vi "vision processing.vi"(0 "Image In":T1, 1 "error in (no error)":errorcluster) -> (2 "error out":errorcluster, 3 "height":dbl, 4 "area":dbl, 5 "x":dbl, 6 "y":dbl, 7 "width":dbl)   [LabVIEW 2011]
uses:
  <vilib>/vision/Image Controls.llb/IMAQ Image.ctl
  fg_typedef.ctl
  <vilib>/vision/NI_Vision_Development_Module.lvlib
panel:
  out "Image Out":T1
  out "error out":errorcluster
  out "Number of Particles Found":i32
  out "Image Out":T1
  out "Number of Hoops Found":i32
  # "0  center of mass x\n1  center of mass y\n2  first pixel x\n3  first pixel y\n4  bounding rect left\n5  bounding rect top\n6  bounding rect right\n7  bounding rect bottom\n8 max feret diameter start x\n9  max feret diameter start y\n10 max feret diameter end x\n11 max feret diameter end y\n12 max horiz segment length left\n13 max horiz segment length right\n14 max horiz segment length row\n15 bounding rect width \n16 bounding rect height\n17 bounding rect diagional\n..\n33 area"
  # "13'3\"\n3'9\""
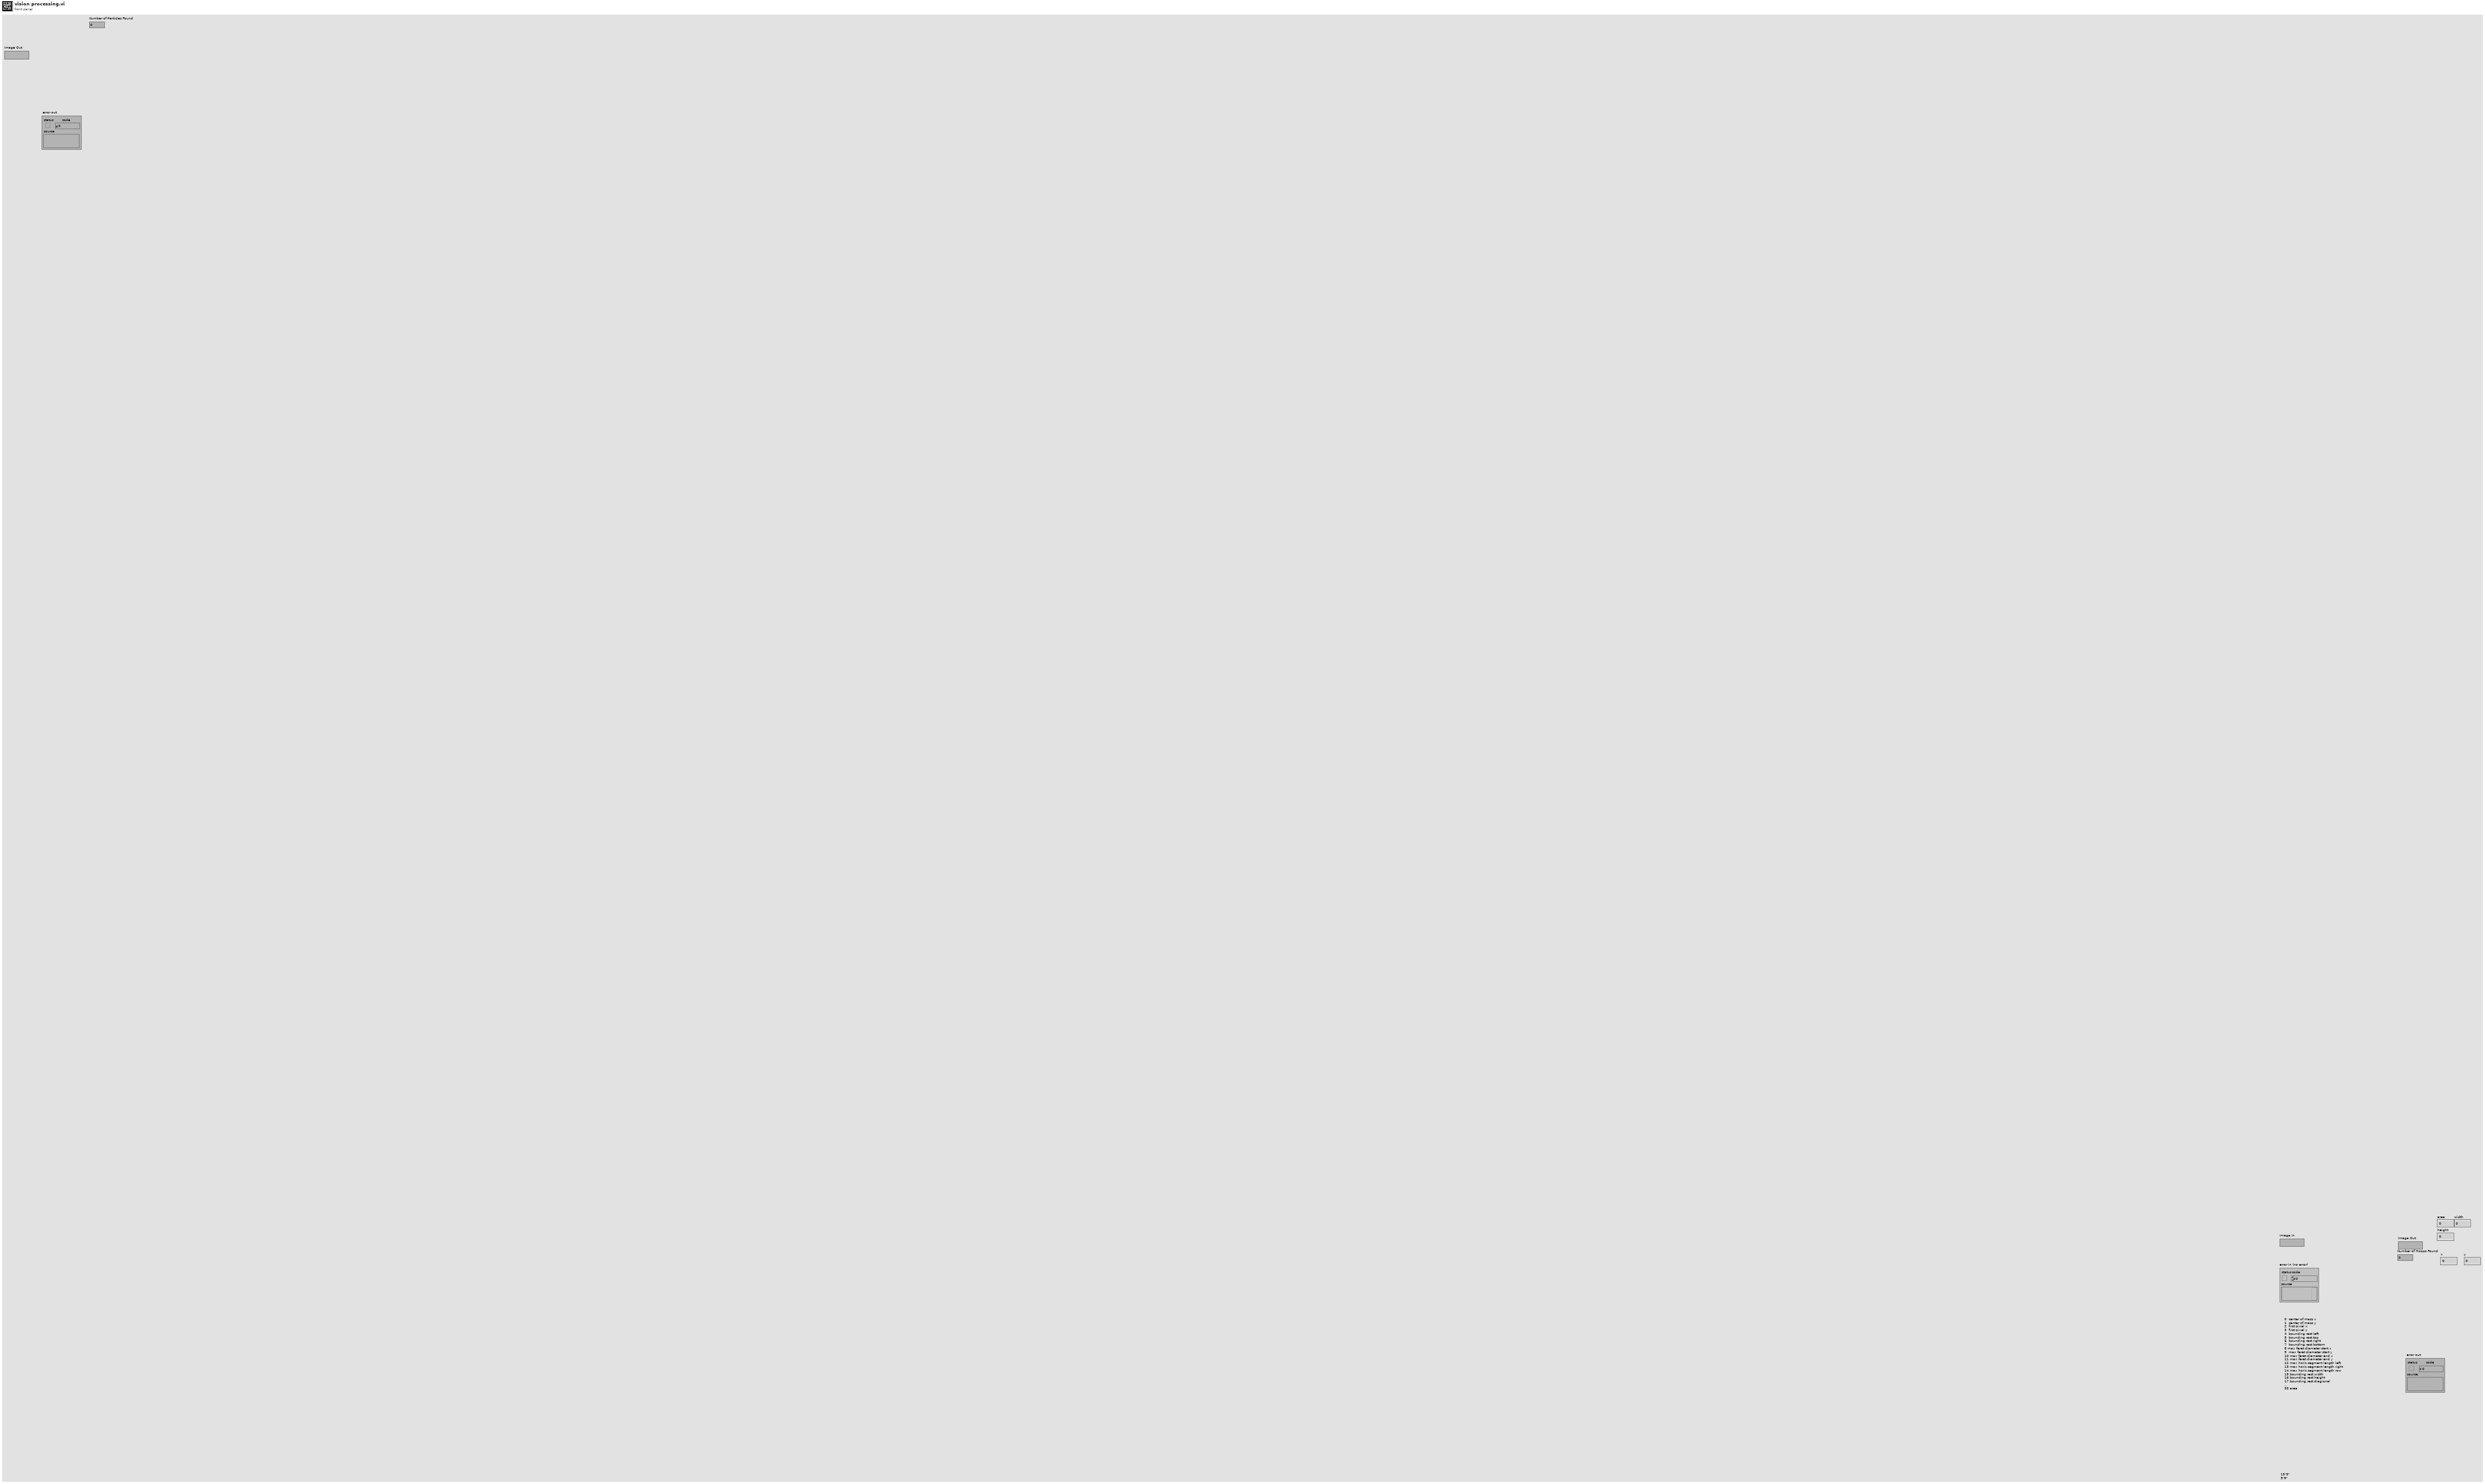
[diagram p1: front panel]
types:
  T1 = typedef "IMAQ Image.ctl" = refnum<image>
  T2 = typedef "Image Type" = u32
  T3 = typedef "fg_typedef.ctl" = enum16{"Get", "Set"}
  T4 = enum32{"AutoM", "Close", "Dilate", "Erode", "Gradient", "Gradient out", "Gradient in", "Hit miss", "Open", "PClose", "POpen", "Thick", "Thin"}
  T5 = cluster{"Brightness":sgl, "Contrast":sgl, "Gamma":sgl}
  T6 = cluster{"Measurement Parameter":i32, "Range Lower Value":dbl, "Range Upper Value":dbl, "Range":bool, "Measurement Type":bool}[]
  T7 = typedef "Particle Parameters" = i32
  T8 = typedef "WPI_DigitalInputDevRef.ctl" = cluster{"DevStatus":errorcluster, "DIO Channel":T9, "Digital Module":T10}
  T9 = typedef "FPGA_DIOChannel.ctl" = enum8{"DIO 1", "DIO 2", "DIO 3", "DIO 4", "DIO 5", "DIO 6", "DIO 7", "DIO 8", "DIO 9", "DIO 10", "DIO 11", "DIO 12", "DIO 13", "DIO 14", "Invalid"}
  T10 = typedef "FPGA_TypedefDigitalModule.ctl" = enum16{"Digital Module 1", "Digital Module 2"}
  T11 = cluster{"Numeric":dbl, "Numeric":dbl, "Numeric":dbl, "Numeric":dbl}
  T12 = cluster{"Numeric":i32, "Numeric":i32, "Numeric":i32, "Numeric":i32}
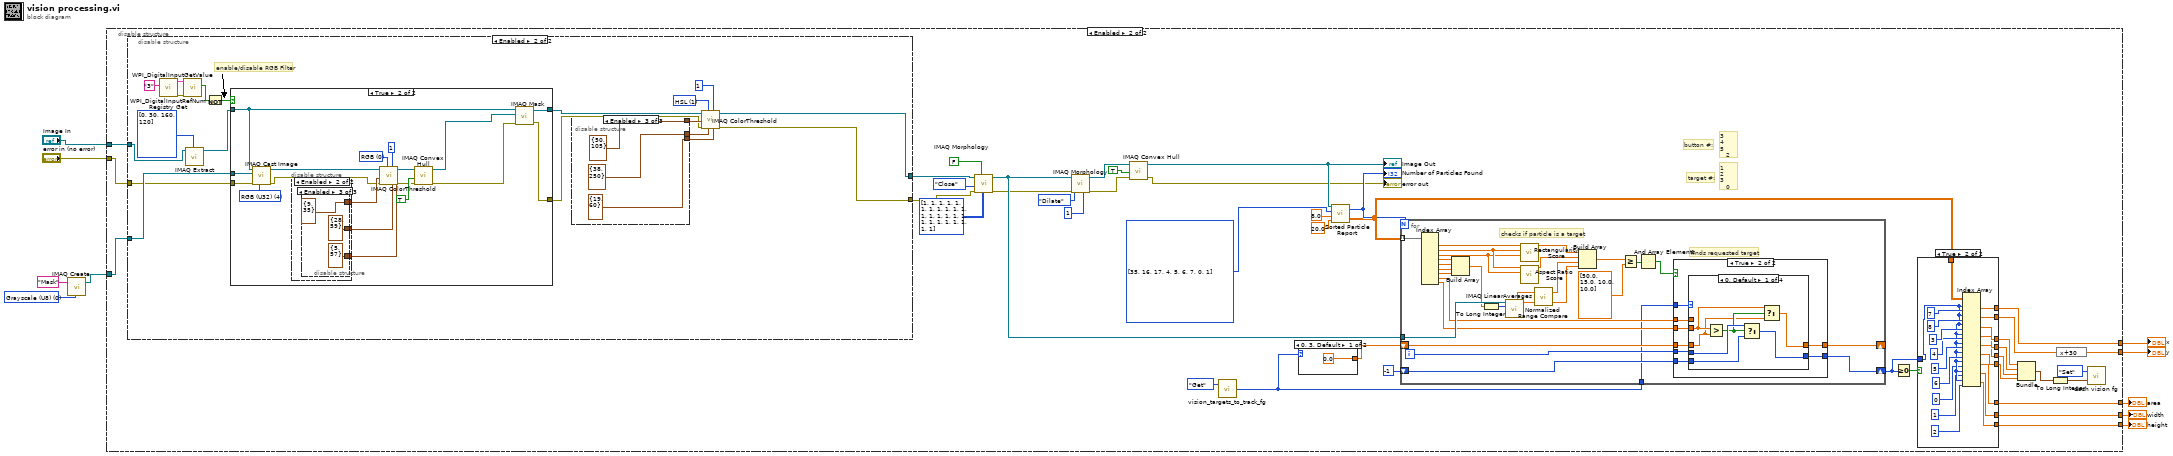
[diagram p0: block diagram]
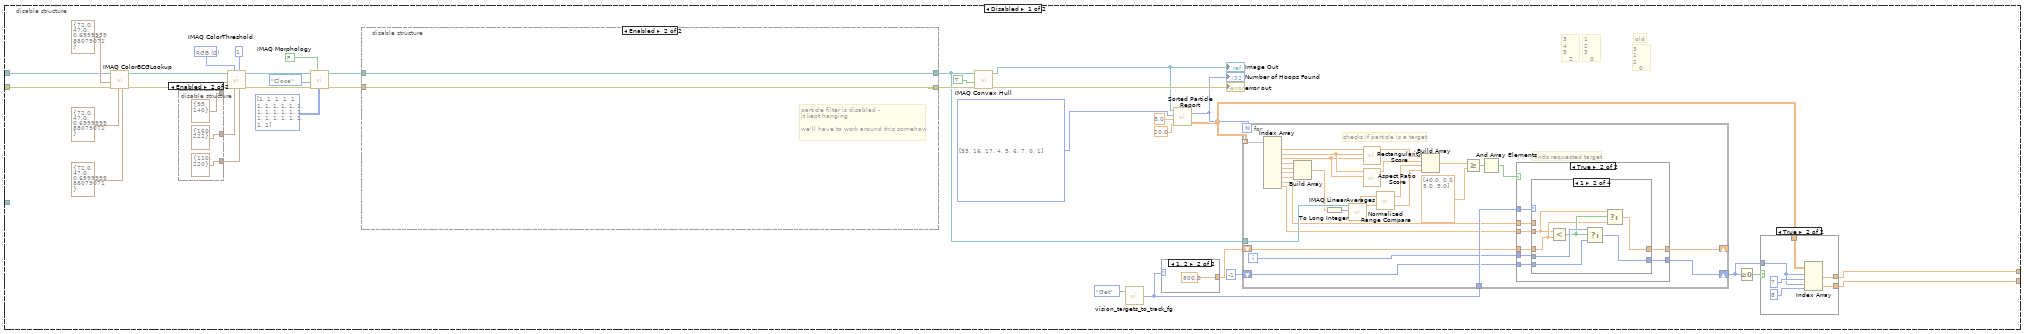
[diagram p2: hidden frame]
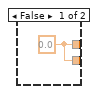
[diagram p3: hidden frame]
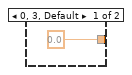
[diagram p4: hidden frame]
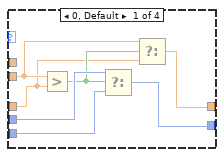
[diagram p6: hidden frame]
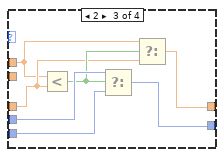
[diagram p7: hidden frame]
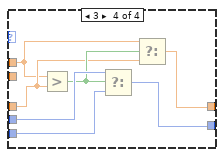
[diagram p8: hidden frame]
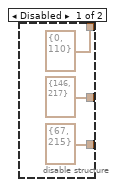
[diagram p9: hidden frame]
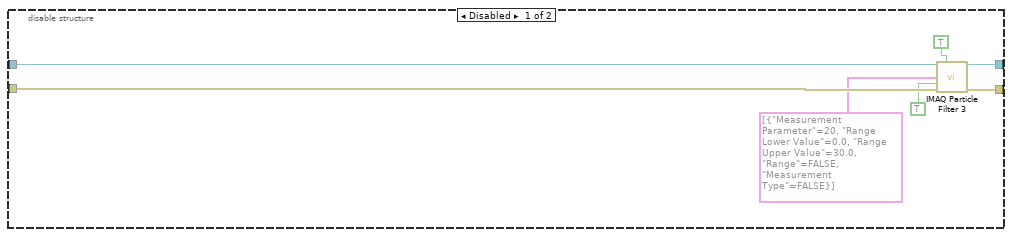
[diagram p10: hidden frame]
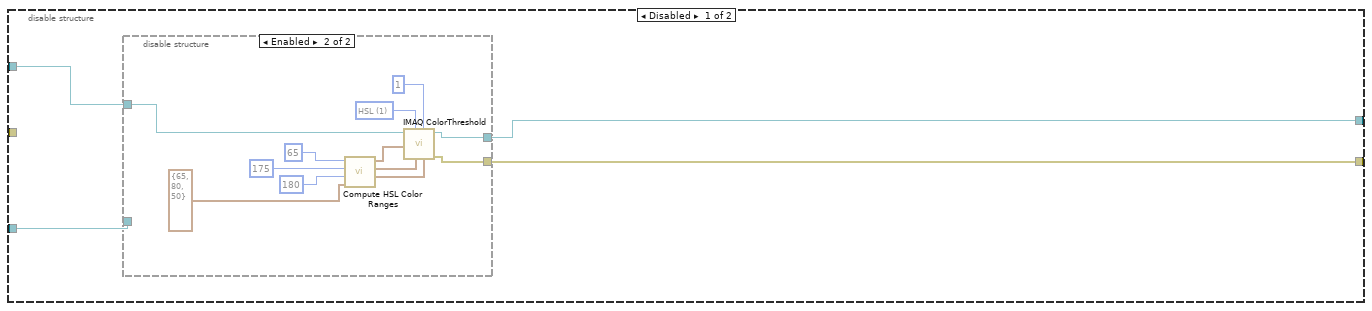
[diagram p11: hidden frame]
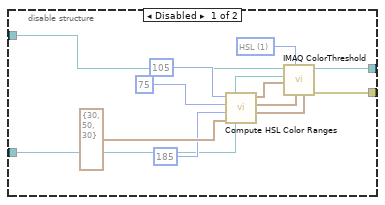
[diagram p12: hidden frame]
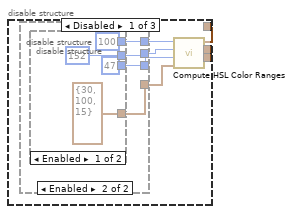
[diagram p13: hidden frame]
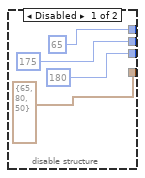
[diagram p14: hidden frame]
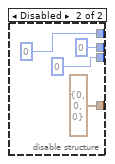
[diagram p15: hidden frame]
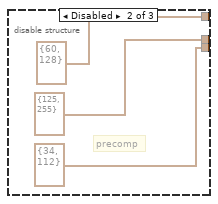
[diagram p16: hidden frame]
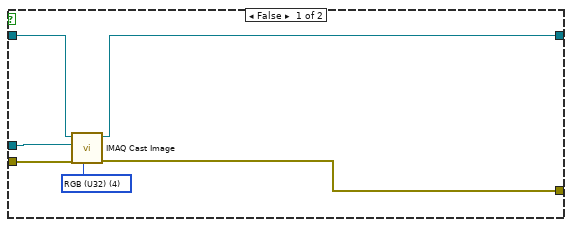
[diagram p17: hidden frame]
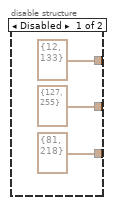
[diagram p18: hidden frame]
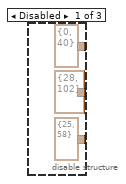
[diagram p19: hidden frame]
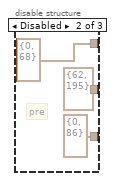
[diagram p20: hidden frame]
diagram:
  w7 = T2 0 items=["Grayscale (U8)", "Grayscale (I16)", "Grayscale (SGL)", "Complex (CSG)", "RGB (U32)", "HSL (U32)", "RGB (U64)", "Grayscale (U16)"] ("Image Type")
  n1 = call "IMAQ Create"("Image Name"="Mask", "Image Type"=w7) -> ("New Image"=w6:T1)  [unwired: 2 in, 2 out]
  n2 = disable-structure shown="Enabled" {
    disable-tunnel: "error in (no error)" -> [w28 w143]
    disable-tunnel: "Image In" -> [w27 w165]
    disable-tunnel: [w13 w162] -> w5
    disable-tunnel: [w12 w139] -> w4
    disable-tunnel: w6 -> [_ w144]
    disable-tunnel: [_ w142] -> w3
    disable-tunnel: [_ w141] -> w2
    disable-tunnel: [_ w140] -> w1
    frame Disabled {
      w20 = T7[] [35, 16, 17, 4, 5, 6, 7, 0, 1] items=["Center of Mass X", "Center of Mass Y", "First Pixel X", "First Pixel Y", "Bounding Rect Left", "Bounding Rect Top", "Bounding Rect Right", "Bounding Rect Bottom", "Max Feret Diameter Start X", "Max Feret Diameter Start Y", "Max Feret Diameter End X", "Max Feret Diameter End Y", "Max Horiz. Segment Length Left", "Max Horiz. Segment Length Right", "Max Horiz. Segment Length Row", "-", "Bounding Rect Width", "Bounding Rect Height", "Bounding Rect Diagonal", "Perimeter", "Convex Hull Perimeter", "Holes' Perimeter", "Max Feret Diameter", "Equivalent Ellipse Major Axis", "Equivalent Ellipse Minor Axis", "Equivalent Ellipse Minor Axis (Feret)", "Equivalent Rect Long Side", "Equivalent Rect Short Side", "Equivalent Rect Diagonal", "Equivalent Rect Short Side (Feret)", "Average Horiz. Segment Length", "Average Vert. Segment Length", "Hydraulic Radius", "Waddel Disk Diameter", "-", "Area", "Holes' Area", "Particle & Holes' Area", "Convex Hull Area", "Image Area", "-", "Number of Holes", "Number of Horiz. Segments", "Number of Vert. Segments", "-", "Orientation", "Max Feret Diameter Orientation", "-", "% Area/Image Area", "% Area/(Particle & Holes' Area)", "Ratio of Equivalent Ellipse Axes", "Ratio of Equivalent Rect Sides", "-", "Elongation Factor", "Compactness Factor", "Heywood Circularity Factor", "Type Factor", "-", "Sum X", "Sum Y", "Sum XX", "Sum XY", "Sum YY", "Sum XXX", "Sum XXY", "Sum XYY", "Sum YYY", "-", "Moment of Inertia XX", "Moment of Inertia XY", "Moment of Inertia YY", "Moment of Inertia XXX", "Moment of Inertia XXY", "Moment of Inertia XYY", "Moment of Inertia YYY", "Norm. Moment of Inertia XX", "Norm. Moment of Inertia XY", "Norm. Moment of Inertia YY", "Norm. Moment of Inertia XXX", "Norm. Moment of Inertia XXY", "Norm. Moment of Inertia XYY", "Norm. Moment of Inertia YYY", "Hu Moment 1", "Hu Moment 2", "Hu Moment 3", "Hu Moment 4", "Hu Moment 5", "Hu Moment 6", "Hu Moment 7"] ("Requested Particle Measurements")
      w42 = u16 0 items=["RGB", "HSL", "HSV", "HSI"] ("Color Mode")
      # "old"
      # "1   \n2     3\n   0"
      # "3   \n1     2\n   0"
      # "3   \n4     5\n   2"
      n3 = call "IMAQ ColorBCGLookup"("Blue BCG Values"=T5 {"Brightness"=72.0, "Contrast"=47.0, "Gamma"=0.7}, "Green BCG Values"=T5 {"Brightness"=72.0, "Contrast"=47.0, "Gamma"=0.7}, "error in (no error)"=w28, "Red BCG Values"=T5 {"Brightness"=72.0, "Contrast"=47.0, "Gamma"=0.7}, "Image Src"=w27) -> ("error out"=w47:errorcluster, "Image Dst Out"=w38:T1)  [unwired: 2 in, 3 out]
      n4 = disable-structure shown="Enabled" {
        disable-tunnel: [cluster{"Lower value":i32, "Upper value":i32} {"Lower value"=0, "Upper value"=110} ("Red or Hue Range") cluster{"Lower value":i32, "Upper value":i32} {"Lower value"=95, "Upper value"=140} ("Red or Hue Range")] -> w41
        disable-tunnel: [cluster{"Lower value":i32, "Upper value":i32} {"Lower value"=146, "Upper value"=217} ("Green or Sat Range") cluster{"Lower value":i32, "Upper value":i32} {"Lower value"=160, "Upper value"=222} ("Green or Sat Range")] -> w40
        disable-tunnel: [cluster{"Lower value":i32, "Upper value":i32} {"Lower value"=67, "Upper value"=215} ("Blue or Luma or Val or Inten Range") cluster{"Lower value":i32, "Upper value":i32} {"Lower value"=110, "Upper value"=220} ("Blue or Luma or Val or Inten Range")] -> w39
        frame Disabled {
        }
        frame Enabled {
        }
      }
      n5 = call "IMAQ ColorThreshold"("Blue or Luma or Val or Inten Range"=w39, "Replace Value"=1, "Green or Sat Range"=w40, "Color Mode"=w42, "error in (no error)"=w47, "Red or Hue Range"=w41, "Image Src"=w38) -> ("error out"=w37:errorcluster, "Image Dst Out"=w33:T1)  [unwired: 1 in, 2 out]
      n6 = call "IMAQ Morphology"("Structuring Element"=i32[][] [[1, 1, 1, 1, 1], [1, 1, 1, 1, 1], [1, 1, 1, 1, 1], [1, 1, 1, 1, 1], [1, 1, 1, 1, 1]], "Square/Hexa (Square)"=FALSE, "error in (no error)"=w37, "Operation"=T4."Close", "Image Src"=w33) -> ("error out"=w32:errorcluster, "Image Dst Out"=w30:T1)  [unwired: 2 in, 3 out]
      n7 = disable-structure shown="Enabled" {
        disable-tunnel: w32 -> [w136 w138]
        disable-tunnel: [w133 w138] -> w31
        disable-tunnel: w30 -> [w132 w137]
        disable-tunnel: [w130 w137] -> w26
        frame Disabled {
          n8 = call "IMAQ Particle Filter 3"("Image Src"=w132, "Connectivity 4/8 (8)"=TRUE, "Selection Values"=T6 [{"Measurement Parameter"=20, "Range Lower Value"=0.0, "Range Upper Value"=30.0, "Range"=FALSE, "Measurement Type"=FALSE}], "Keep/Remove Particles (F)"=TRUE ("Keep/Remove Particles"), "error in (no error)"=w136) -> ("Image Dst Out"=w130:T1, "error out"=w133:errorcluster)  [unwired: 4 in, 5 out]
        }
        frame Enabled {
          # "particle filter is disabled - \nit kept hanging\n\nwe'll have to work around this somehow"
        }
      }
      n9 = call "IMAQ Convex Hull"("error in (no error)"=w31, "Connectivity 4/8 (8)"=TRUE, "Image Src"=w26) -> ("error out"=→"error out":errorcluster, "Image Dst Out"=w11:T1)  [unwired: 1 in, 6 out]
      "Image Out" <- w11
      n10 = call "vision_targets_to_track_fg.vi"("Menu (Get)"=fg_typedef."Get") -> ("Output"=w23:i32)  [unwired: 1 in]
      n11 = case shown="1, 2" w23 {
        tunnel: [0.0 ("element") 800.0 ("element")] -> w24
        frame 0, 3, Default {
        }
        frame 1, 2 {
        }
      }
      n12 = call "Sorted Particle Report.vi"("Area Size Limit"=20.0, "Particle Count Limit"=8.0, "Pixel Measurements"=w20, "Image in"=w11) -> ("Sorted Data"=w16:dbl[][], "Particles"=w17:i32)
      "Number of Hoops Found" <- w17
      n13 = for {
        N: w17 -> [_]
        tunnel: w26 -> [w85]
        tunnel: w16 -> [w84] mode=indexing
        tunnel: w23 -> [w74]
        shift-right: [w66] -> _
        shift-left: w24 -> [w69]
        shift-right: [w67] -> w15
        shift-left: -1 -> [w68]
        i -> [w70]
        # "checks if particle is a target"
        # "finds requested target"
        n14 = Index Array(array=w84) -> (element #1=w65:dbl, element #2=w62:dbl, element #3=w61:dbl, element #4=w80:dbl, element #5=w79:dbl, element #6=w78:dbl, element #7=w77:dbl, element #8=w72:dbl, element #9=w73:dbl)  [unwired: 9 in]
        n15 = Build Array(w80, w79, w78, w77) -> (w76:dbl[])
        n16 = To Long Integer(number=w76) -> (32bit integer=w75:i32[])
        n17 = call "IMAQ LinearAverages"("Optional Rectangle"=w75, "Image Src"=w85) -> ("Y Axis Averages"=w57:sgl[], "X Axis Averages"=w58:sgl[])  [unwired: 2 in, 6 out]
        n18 = call "Rectangularity Score.vi"("Height"=w61, "Width"=w62, "Area"=w65) -> ("Score"=w64:dbl)  [unwired: 8 in]
        n19 = call "Aspect Ratio Score.vi"("Height"=w61, "Width"=w62) -> ("Score"=w63:dbl)  [unwired: 9 in]
        n20 = call "Normalized Range Compare.vi"("Y Averages"=w57, "X Averages"=w58) -> ("Y Score"=w59:dbl, "X Score"=w60:dbl)
        n21 = Build Array(w64, w63, w60, w59) -> (w83:dbl[])
        n22 = Greater Or Equal?(x=w83, y=dbl[] [40.0, 0.0, 5.0, 5.0]) -> (x >= y?=w81:bool[])
        n23 = And Array Elements(Boolean array=w81) -> (logical AND=w71:bool)
        n24 = case shown="True" w71 {
          tunnel: w74 -> [_ w95]
          tunnel: w73 -> [_ w94]
          tunnel: w72 -> [_ w93]
          tunnel: w70 -> [_ w92]
          tunnel: w69 -> [w86 w91]
          tunnel: w68 -> [w87 w90]
          tunnel: [w87 w89] -> w67
          tunnel: [w86 w88] -> w66
          frame False {
          }
          frame True {
            n25 = case shown="1" w95 {
              tunnel: w94 -> [w98 w103 _ _]
              tunnel: w93 -> [_ _ w110 w117]
              tunnel: w92 -> [w102 w109 w116 w123]
              tunnel: w91 -> [w97 w105 w112 w119]
              tunnel: w90 -> [w101 w108 w115 w122]
              tunnel: [w100 w107 w114 w121] -> w89
              tunnel: [w96 w104 w111 w118] -> w88
              frame 0, Default {
                n26 = Greater?(x=w98, y=w97) -> (0:w99:bool)
                n27 = Select(t=w102, s=w99, f=w101) -> (s? t:f=w100:i32)
                n28 = Select(t=w98, s=w99, f=w97) -> (s? t:f=w96:dbl)
              }
              frame 1 {
                n29 = Less?(x=w103, y=w105) -> (x < y?=w106:bool)
                n30 = Select(t=w109, s=w106, f=w108) -> (s? t:f=w107:i32)
                n31 = Select(t=w103, s=w106, f=w105) -> (s? t:f=w104:dbl)
              }
              frame 2 {
                n32 = Less?(x=w110, y=w112) -> (x < y?=w113:bool)
                n33 = Select(t=w116, s=w113, f=w115) -> (s? t:f=w114:i32)
                n34 = Select(t=w110, s=w113, f=w112) -> (s? t:f=w111:dbl)
              }
              frame 3 {
                n35 = Greater?(x=w117, y=w119) -> (0:w120:bool)
                n36 = Select(t=w123, s=w120, f=w122) -> (s? t:f=w121:i32)
                n37 = Select(t=w117, s=w120, f=w119) -> (s? t:f=w118:dbl)
              }
            }
          }
        }
      }
      n38 = Greater Or Equal To 0?(x=w15) -> (x >= 0?=w14:bool)
      n39 = case shown="True" w14 {
        tunnel: [w48 w52] -> w13
        tunnel: [w48 w51] -> w12
        tunnel: w16 -> [_ w50]
        tunnel: w15 -> [_ w49]
        frame False {
          w48 = 0.0 ("Numeric")
        }
        frame True {
          n40 = Index Array(array=w50, index (row) #1=w49, index (col) #1=7, index (row) #2=w49, index (col) #2=8) -> (element #1=w52:dbl, element #2=w51:dbl)
        }
      }
    }
    frame Enabled {
      w164 = T7[] [35, 16, 17, 4, 5, 6, 7, 0, 1] items=["Center of Mass X", "Center of Mass Y", "First Pixel X", "First Pixel Y", "Bounding Rect Left", "Bounding Rect Top", "Bounding Rect Right", "Bounding Rect Bottom", "Max Feret Diameter Start X", "Max Feret Diameter Start Y", "Max Feret Diameter End X", "Max Feret Diameter End Y", "Max Horiz. Segment Length Left", "Max Horiz. Segment Length Right", "Max Horiz. Segment Length Row", "-", "Bounding Rect Width", "Bounding Rect Height", "Bounding Rect Diagonal", "Perimeter", "Convex Hull Perimeter", "Holes' Perimeter", "Max Feret Diameter", "Equivalent Ellipse Major Axis", "Equivalent Ellipse Minor Axis", "Equivalent Ellipse Minor Axis (Feret)", "Equivalent Rect Long Side", "Equivalent Rect Short Side", "Equivalent Rect Diagonal", "Equivalent Rect Short Side (Feret)", "Average Horiz. Segment Length", "Average Vert. Segment Length", "Hydraulic Radius", "Waddel Disk Diameter", "-", "Area", "Holes' Area", "Particle & Holes' Area", "Convex Hull Area", "Image Area", "-", "Number of Holes", "Number of Horiz. Segments", "Number of Vert. Segments", "-", "Orientation", "Max Feret Diameter Orientation", "-", "% Area/Image Area", "% Area/(Particle & Holes' Area)", "Ratio of Equivalent Ellipse Axes", "Ratio of Equivalent Rect Sides", "-", "Elongation Factor", "Compactness Factor", "Heywood Circularity Factor", "Type Factor", "-", "Sum X", "Sum Y", "Sum XX", "Sum XY", "Sum YY", "Sum XXX", "Sum XXY", "Sum XYY", "Sum YYY", "-", "Moment of Inertia XX", "Moment of Inertia XY", "Moment of Inertia YY", "Moment of Inertia XXX", "Moment of Inertia XXY", "Moment of Inertia XYY", "Moment of Inertia YYY", "Norm. Moment of Inertia XX", "Norm. Moment of Inertia XY", "Norm. Moment of Inertia YY", "Norm. Moment of Inertia XXX", "Norm. Moment of Inertia XXY", "Norm. Moment of Inertia XYY", "Norm. Moment of Inertia YYY", "Hu Moment 1", "Hu Moment 2", "Hu Moment 3", "Hu Moment 4", "Hu Moment 5", "Hu Moment 6", "Hu Moment 7"] ("Requested Particle Measurements")
      # "target #:"
      # "button #:"
      # "1   \n2     3\n   0"
      # "3   \n4     5\n   2"
      n41 = disable-structure shown="Enabled" {
        disable-tunnel: [w183 w216] -> w176
        disable-tunnel: [w182 w217] -> w175
        disable-tunnel: w165 -> [w181 w209]
        disable-tunnel: w144 -> [w180 w226]
        disable-tunnel: w143 -> [_ w225]
        frame Disabled {
          n42 = disable-structure shown="Enabled" {
            disable-tunnel: [w195 w198] -> w183
            disable-tunnel: [w194 w199] -> w182
            disable-tunnel: w181 -> [w185 w197]
            disable-tunnel: w180 -> [w184 _]
            frame Disabled {
              w193 = u16 1 items=["RGB", "HSL", "HSV", "HSI"] ("Color Mode")
              n43 = call "Compute HSL Color Ranges.vi"("Margins"=cluster{"Hue":i32, "Sat":i32, "Lum":i32} {"Hue"=30, "Sat"=50, "Lum"=30}, "Luminance"=185, "Saturation"=75, "Hue"=105) -> ("Lum Range"=w190:cluster{i32, i32}, "Sat Range"=w191:cluster{i32, i32}, "Hue Range"=w192:cluster{i32, i32})  [unwired: 5 in]
              n44 = call "IMAQ ColorThreshold"("Blue or Luma or Val or Inten Range"=w190, "Green or Sat Range"=w191, "Color Mode"=w193, "Red or Hue Range"=w192, "Image Dst"=w184, "Image Src"=w185) -> ("error out"=w195:errorcluster, "Image Dst Out"=w194:T1)  [unwired: 4 in]
            }
            frame Enabled {
              w201 = u16 1 items=["RGB", "HSL", "HSV", "HSI"] ("Color Mode")
              n45 = call "Compute HSL Color Ranges.vi"("Margins"=cluster{"Hue":i32, "Sat":i32, "Lum":i32} {"Hue"=65, "Sat"=80, "Lum"=50}, "Luminance"=180, "Saturation"=175, "Hue"=65) -> ("Lum Range"=w204:cluster{i32, i32}, "Sat Range"=w203:cluster{i32, i32}, "Hue Range"=w202:cluster{i32, i32})  [unwired: 5 in]
              n46 = call "IMAQ ColorThreshold"("Blue or Luma or Val or Inten Range"=w204, "Replace Value"=1, "Green or Sat Range"=w203, "Color Mode"=w201, "Red or Hue Range"=w202, "Image Src"=w197) -> ("error out"=w198:errorcluster, "Image Dst Out"=w199:T1)  [unwired: 4 in]
            }
          }
        }
        frame Enabled {
          w221 = u16 1 items=["RGB", "HSL", "HSV", "HSI"] ("Color Mode")
          # "enable/disable RGB Filter"
          n47 = call <vilib>:"WPI_DigitalInputRefNum Registry Get.vi"("refnum name"="3") -> ("error out"=w214:errorcluster, "DigitalInputDevRef"=w215:T8)  [unwired: 9 in]
          n48 = call <vilib>:"WPI_DigitalInputGetValue.vi"("error in (no error)"=w214, "DigitalInputDevRef"=w215) -> ("Value"=w212:bool)  [unwired: 7 in, 2 out]
          n49 = call "IMAQ Extract"("Optional Rectangle"=i32[] [0, 30, 160, 120], "Image Src"=w209) -> ("Image Dst Out"=w208:T1)  [unwired: 8 in, 1 out]
          n50 = Not(x=w212) -> (.not. x?=w211:bool)
          n51 = case shown="True" w211 {
            tunnel: [w258 w279] -> w219
            tunnel: w226 -> [w260 w271]
            tunnel: w208 -> [w259 w270]
            tunnel: [w257 w266] -> w218
            tunnel: w225 -> [w256 w263]
            frame False {
              w261 = T2 4 items=["Grayscale (U8)", "Grayscale (I16)", "Grayscale (SGL)", "Complex (CSG)", "RGB (U32)", "HSL (U32)", "RGB (U64)"] ("Image Type")
              n52 = call "IMAQ Cast Image"("Image Type"=w261, "error in (no error)"=w256, "Image Dst"=w260, "Image Src"=w259) -> ("error out"=w257:errorcluster, "Image Dst Out"=w258:T1)  [unwired: 6 in]
            }
            frame True {
              w276 = u16 0 items=["RGB", "HSL", "HSV", "HSI"] ("Color Mode")
              w278 = T2 4 items=["Grayscale (U8)", "Grayscale (I16)", "Grayscale (SGL)", "Complex (CSG)", "RGB (U32)", "HSL (U32)", "RGB (U64)"] ("Image Type")
              n53 = call "IMAQ Cast Image"("Image Type"=w278, "error in (no error)"=w263, "Image Dst"=w271, "Image Src"=w270) -> ("error out"=w264:errorcluster, "Image Dst Out"=w274:T1)  [unwired: 6 in]
              n54 = disable-structure shown="Enabled" {
                disable-tunnel: [cluster{"Lower value":i32, "Upper value":i32} {"Lower value"=12, "Upper value"=133} ("Red or Hue Range") w285] -> w268
                disable-tunnel: [cluster{"Lower value":i32, "Upper value":i32} {"Lower value"=127, "Upper value"=255} ("Green or Sat Range") w284] -> w267
                disable-tunnel: [cluster{"Lower value":i32, "Upper value":i32} {"Lower value"=81, "Upper value"=218} ("Blue or Luma or Val or Inten Range") w283] -> w262
                frame Disabled {
                }
                frame Enabled {
                  n55 = disable-structure shown="Enabled" {
                    disable-tunnel: [cluster{"Lower value":i32, "Upper value":i32} {"Lower value"=0, "Upper value"=40} ("Red or Hue Range") cluster{"Lower value":i32, "Upper value":i32} {"Lower value"=0, "Upper value"=68} ("Red or Hue Range") cluster{"Lower value":i32, "Upper value":i32} {"Lower value"=9, "Upper value"=35} ("Red or Hue Range")] -> w285
                    disable-tunnel: [cluster{"Lower value":i32, "Upper value":i32} {"Lower value"=28, "Upper value"=102} ("Green or Sat Range") cluster{"Lower value":i32, "Upper value":i32} {"Lower value"=62, "Upper value"=195} ("Green or Sat Range") cluster{"Lower value":i32, "Upper value":i32} {"Lower value"=28, "Upper value"=59} ("Green or Sat Range")] -> w284
                    disable-tunnel: [cluster{"Lower value":i32, "Upper value":i32} {"Lower value"=25, "Upper value"=58} ("Blue or Luma or Val or Inten Range") cluster{"Lower value":i32, "Upper value":i32} {"Lower value"=0, "Upper value"=86} ("Blue or Luma or Val or Inten Range") cluster{"Lower value":i32, "Upper value":i32} {"Lower value"=5, "Upper value"=57} ("Blue or Luma or Val or Inten Range")] -> w283
                    frame Disabled {
                    }
                    frame Disabled {
                      # "pre"
                    }
                    frame Enabled {
                    }
                  }
                }
              }
              n56 = call "IMAQ ColorThreshold"("Blue or Luma or Val or Inten Range"=w262, "Replace Value"=1, "Green or Sat Range"=w267, "Color Mode"=w276, "error in (no error)"=w264, "Red or Hue Range"=w268, "Image Src"=w274) -> ("error out"=w272:errorcluster, "Image Dst Out"=w273:T1)  [unwired: 1 in, 2 out]
              n57 = call "IMAQ Convex Hull"("error in (no error)"=w272, "Connectivity 4/8 (8)"=TRUE, "Image Src"=w273) -> ("error out"=w265:errorcluster, "Image Dst Out"=w269:T1)  [unwired: 7 in]
              n58 = call "IMAQ Mask"("error in (no error)"=w265, "Image Mask"=w269, "Image Src"=w270) -> ("error out"=w266:errorcluster, "Image Dst Out"=w279:T1)  [unwired: 2 in]
            }
          }
          n59 = disable-structure shown="Enabled" {
            disable-tunnel: [w229 cluster{"Lower value":i32, "Upper value":i32} {"Lower value"=34, "Upper value"=112} ("Blue or Luma or Val or Inten Range") cluster{"Lower value":i32, "Upper value":i32} {"Lower value"=19, "Upper value"=60} ("Blue or Luma or Val or Inten Range")] -> w224
            disable-tunnel: [w228 cluster{"Lower value":i32, "Upper value":i32} {"Lower value"=125, "Upper value"=255} ("Green or Sat Range") cluster{"Lower value":i32, "Upper value":i32} {"Lower value"=38, "Upper value"=250} ("Green or Sat Range")] -> w223
            disable-tunnel: [w227 cluster{"Lower value":i32, "Upper value":i32} {"Lower value"=60, "Upper value"=128} ("Red or Hue Range") cluster{"Lower value":i32, "Upper value":i32} {"Lower value"=50, "Upper value"=105} ("Red or Hue Range")] -> w222
            frame Disabled {
              n60 = disable-structure shown="Enabled" {
                disable-tunnel: [65 ("Hue") w241] -> w233
                disable-tunnel: [175 ("Saturation") w240] -> w232
                disable-tunnel: [180 ("Luminance") w239] -> w231
                disable-tunnel: [cluster{"Hue":i32, "Sat":i32, "Lum":i32} {"Hue"=65, "Sat"=80, "Lum"=50} ("Margins") w238] -> w230
                frame Disabled {
                }
                frame Enabled {
                  n61 = disable-structure shown="Enabled" {
                    disable-tunnel: [100 ("Hue") 0 ("Hue")] -> w241
                    disable-tunnel: [152 ("Saturation") 0 ("Saturation")] -> w240
                    disable-tunnel: [47 ("Luminance") 0 ("Luminance")] -> w239
                    disable-tunnel: [cluster{"Hue":i32, "Sat":i32, "Lum":i32} {"Hue"=30, "Sat"=100, "Lum"=15} ("Margins") cluster{"Hue":i32, "Sat":i32, "Lum":i32} {"Hue"=0, "Sat"=0, "Lum"=0} ("Margins")] -> w238
                    frame Enabled {
                    }
                    frame Disabled {
                    }
                  }
                }
              }
              n62 = call "Compute HSL Color Ranges.vi"("Margins"=w230, "Luminance"=w231, "Saturation"=w232, "Hue"=w233) -> ("Lum Range"=w229:cluster{i32, i32}, "Sat Range"=w228:cluster{i32, i32}, "Hue Range"=w227:cluster{i32, i32})  [unwired: 5 in]
            }
            frame Disabled {
              # "precomp"
            }
            frame Enabled {
            }
          }
          n63 = call "IMAQ ColorThreshold"("Blue or Luma or Val or Inten Range"=w224, "Replace Value"=1, "Green or Sat Range"=w223, "Color Mode"=w221, "error in (no error)"=w218, "Red or Hue Range"=w222, "Image Src"=w219) -> ("error out"=w216:errorcluster, "Image Dst Out"=w217:T1)  [unwired: 3 in]
        }
      }
      n64 = call "IMAQ Morphology"("Structuring Element"=i32[][] [[1, 1, 1, 1, 1], [1, 1, 1, 1, 1], [1, 1, 1, 1, 1], [1, 1, 1, 1, 1], [1, 1, 1, 1, 1]], "Square/Hexa (Square)"=FALSE, "error in (no error)"=w176, "Operation"=T4."Close", "Image Src"=w175) -> ("error out"=w154:errorcluster, "Image Dst Out"=w156:T1)  [unwired: 2 in, 3 out]
      n65 = call "IMAQ Morphology"("Number of iterations (1)"=1, "error in (no error)"=w154, "Operation"=T4."Dilate", "Image Src"=w156) -> ("error out"=w153:errorcluster, "Image Dst Out"=w155:T1)  [unwired: 6 in]
      n66 = call "IMAQ Convex Hull"("error in (no error)"=w153, "Connectivity 4/8 (8)"=TRUE, "Image Src"=w155) -> ("error out"=→"error out":errorcluster, "Image Dst Out"=w163:T1)  [unwired: 1 in, 6 out]
      "Image Out" <- w163
      n67 = call "vision_targets_to_track_fg.vi"("Menu (Get)"=fg_typedef."Get") -> ("Output"=w159:i32)  [unwired: 1 in]
      n68 = case shown="0, 3, Default" w159 {
        tunnel: [0.0 ("element") 800.0 ("element")] -> w173
        frame 0, 3, Default {
        }
        frame 1, 2 {
        }
      }
      n69 = call "Sorted Particle Report.vi"("Area Size Limit"=20.0, "Particle Count Limit"=8.0, "Pixel Measurements"=w164, "Image in"=w163) -> ("Sorted Data"=w168:dbl[][], "Particles"=w172:i32)
      "Number of Particles Found" <- w172
      n70 = for {
        N: w172 -> [_]
        tunnel: w156 -> [w346]
        tunnel: w168 -> [w345] mode=indexing
        shift-right: [w328] -> _
        shift-left: w173 -> [w331]
        shift-right: [w329] -> w167
        shift-left: -1 -> [w330]
        tunnel: w159 -> [w318]
        i -> [w332]
        # "checks if particle is a target"
        # "finds requested target"
        n71 = Index Array(array=w345) -> (element #1=w327:dbl, element #2=w324:dbl, element #3=w323:dbl, element #4=w341:dbl, element #5=w340:dbl, element #6=w339:dbl, element #7=w338:dbl, element #8=w334:dbl, element #9=w335:dbl)  [unwired: 9 in]
        n72 = Build Array(w341, w340, w339, w338) -> (w337:dbl[])
        n73 = To Long Integer(number=w337) -> (32bit integer=w336:i32[])
        n74 = call "IMAQ LinearAverages"("Optional Rectangle"=w336, "Image Src"=w346) -> ("Y Axis Averages"=w319:sgl[], "X Axis Averages"=w320:sgl[])  [unwired: 2 in, 6 out]
        n75 = call "Rectangularity Score.vi"("Height"=w323, "Width"=w324, "Area"=w327) -> ("Score"=w326:dbl)  [unwired: 8 in]
        n76 = call "Aspect Ratio Score.vi"("Height"=w323, "Width"=w324) -> ("Score"=w325:dbl)  [unwired: 9 in]
        n77 = call "Normalized Range Compare.vi"("Y Averages"=w319, "X Averages"=w320) -> ("Y Score"=w321:dbl, "X Score"=w322:dbl)
        n78 = Build Array(w326, w325, w322, w321) -> (w344:dbl[])
        n79 = Greater Or Equal?(x=w344, y=dbl[] [50.0, 15.0, 10.0, 10.0]) -> (x >= y?=w342:bool[])
        n80 = And Array Elements(Boolean array=w342) -> (logical AND=w333:bool)
        n81 = case shown="True" w333 {
          tunnel: w335 -> [_ w356]
          tunnel: w334 -> [_ w355]
          tunnel: w332 -> [_ w354]
          tunnel: w331 -> [w347 w353]
          tunnel: w330 -> [w348 w352]
          tunnel: [w348 w351] -> w329
          tunnel: [w347 w350] -> w328
          tunnel: w318 -> [_ w349]
          frame False {
          }
          frame True {
            n82 = case shown="0, Default" w349 {
              tunnel: w356 -> [w359 w364 _ _]
              tunnel: w355 -> [_ _ w371 w378]
              tunnel: w354 -> [w363 w370 w377 w384]
              tunnel: w353 -> [w358 w366 w373 w380]
              tunnel: w352 -> [w362 w369 w376 w383]
              tunnel: [w361 w368 w375 w382] -> w351
              tunnel: [w357 w365 w372 w379] -> w350
              frame 0, Default {
                n83 = Greater?(x=w359, y=w358) -> (0:w360:bool)
                n84 = Select(t=w363, s=w360, f=w362) -> (s? t:f=w361:i32)
                n85 = Select(t=w359, s=w360, f=w358) -> (s? t:f=w357:dbl)
              }
              frame 1 {
                n86 = Less?(x=w364, y=w366) -> (x < y?=w367:bool)
                n87 = Select(t=w370, s=w367, f=w369) -> (s? t:f=w368:i32)
                n88 = Select(t=w364, s=w367, f=w366) -> (s? t:f=w365:dbl)
              }
              frame 2 {
                n89 = Less?(x=w371, y=w373) -> (x < y?=w374:bool)
                n90 = Select(t=w377, s=w374, f=w376) -> (s? t:f=w375:i32)
                n91 = Select(t=w371, s=w374, f=w373) -> (s? t:f=w372:dbl)
              }
              frame 3 {
                n92 = Greater?(x=w378, y=w380) -> (0:w381:bool)
                n93 = Select(t=w384, s=w381, f=w383) -> (s? t:f=w382:i32)
                n94 = Select(t=w378, s=w381, f=w380) -> (s? t:f=w379:dbl)
              }
            }
          }
        }
      }
      n95 = Greater Or Equal To 0?(x=w167) -> (x >= 0?=w166:bool)
      n96 = case shown="True" w166 {
        tunnel: [w297 w315] -> w162
        tunnel: [w297 w314] -> w161
        tunnel: w168 -> [_ w313]
        tunnel: w167 -> [_ w304]
        tunnel: [w297 w308] -> w150
        tunnel: [w297 w307] -> w149
        tunnel: [w297 w306] -> w148
        tunnel: [w297 w305] -> w147
        tunnel: [w297 w300] -> w142
        tunnel: [w297 w299] -> w141
        tunnel: [w297 w298] -> w140
        frame False {
          w297 = 0.0 ("Numeric")
        }
        frame True {
          n97 = Index Array(array=w313, index (row) #1=w304, index (col) #1=7, index (row) #2=w304, index (col) #2=8, index (row) #3=w304, index (col) #3=3, index (row) #4=w304, index (col) #4=4, index (row) #5=w304, index (col) #5=5, index (row) #6=w304, index (col) #6=6, index (row) #7=w304, index (col) #7=0, index (row) #8=w304, index (col) #8=1, index (row) #9=w304, index (col) #9=2) -> (element #1=w315:dbl, element #2=w314:dbl, element #3=w308:dbl, element #4=w307:dbl, element #5=w306:dbl, element #6=w305:dbl, element #7=w300:dbl, element #8=w299:dbl, element #9=w298:dbl)
        }
      }
      n98 = Bundle("Numeric"=w150, "Numeric"=w149, "Numeric"=w148, "Numeric"=w147) -> (w146:T11)  [unwired: 1 in]
      n99 = To Long Integer(number=w146) -> (32bit integer=w145:T12)
      n100 = expression code="x+30"(w161) -> (w139:dbl)
      n101 = call "dash vision fg.vi"("Input"=w145, "Menu"=fg_typedef."Set") -> ()  [unwired: 1 out]
    }
  }
  "x" <- w5
  "y" <- w4
  "area" <- w3
  "width" <- w2
  "height" <- w1
